vi "APU Synchronization Trigger.vi"(6 "trigger line.<user name>":refnum<k21>="PXI_Trig0", 11 "send trigger.<user name>":bool) -> ()   [LabVIEW 2015, in "Engine Simulation Toolkit.lvlib" / "APU.lvlib"]
uses:
  APU.lvlib
  <vilib>/rvi/eio/common/nirviEmuTemplateMethod_errors.vi
  <vilib>/eio/EIOMethodNode/EIOMethodNode.xnode
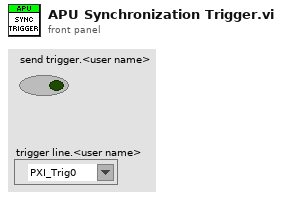
[diagram p1: front panel]
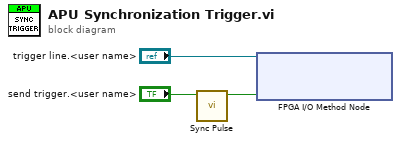
[diagram p0: block diagram]
diagram:
  n1 = call "Sync Pulse.vi"("Sync"="send trigger.<user name>") -> ("Sync Enable?"=w1:bool)  [unwired: 10 in]
  n2 = xnode "FPGA I/O Method Node"("FPGA I/O In"="trigger line.<user name>", "Enable"=w1) -> ()  [unwired: 1 out]
